vi "ALTS-2015 Check Serial Number Empty.vi"(8 "error in (no error)":errorcluster, 11 "Serial Number":string) -> (0 "error out":errorcluster, 2 "SN Empty?":bool, 3 "Serial Number out":string)   [LabVIEW 2013]
doc: "Copyright © 2005, Soliton Technologies.\nAll rights reserved."
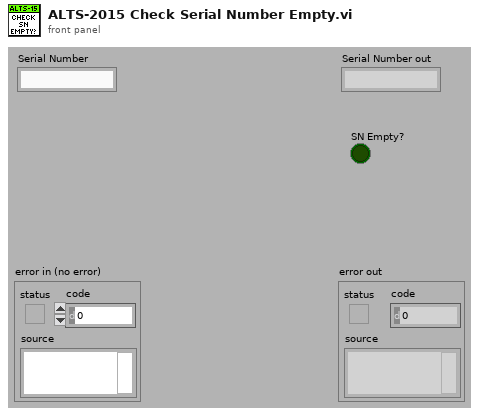
[diagram p1: front panel]
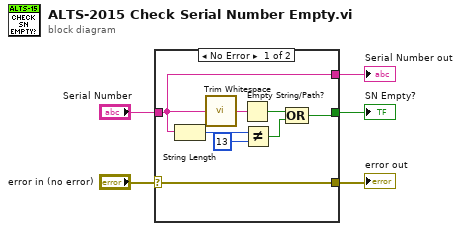
[diagram p0: block diagram]
diagram:
  n1 = case shown="No Error" "error in (no error)" {
    selector: "error in (no error)" -> [w13 w16]
    tunnel: [w13 w16] -> w4
    tunnel: "Serial Number" -> [w8 _]
    tunnel: [w8 "" ("Serial Number")] -> w2
    tunnel: [w12 FALSE] -> w1
    frame No Error {
      n2 = String Length(string=w8) -> (length=w10:i32)
      n3 = call <vilib>:"Trim Whitespace.vi"("string"=w8) -> ("trimmed string"=w9:string)  [unwired: 1 in]
      n4 = Empty String/Path?(string/path=w9) -> (empty?=w7:bool)
      n5 = Not Equal?(x=w10, y=13) -> (x != y?=w6:bool)
      n6 = Compound Arithmetic op=OR(w7, w6) -> (w12:bool)
    }
    frame Error {
    }
  }
  "error out" <- w4
  "Serial Number out" <- w2
  "SN Empty?" <- w1
